vi "Get Call Result.vi"(8 "error in (no error)":errorcluster, 11 "Response body":string) -> (0 "error out":errorcluster, 3 "Call Result":string)   [LabVIEW 2015, in "AWS Core.lvlib"]
uses:
  AWS Core.lvlib
  <vilib>/regexp/Match Regular Expression.xnode
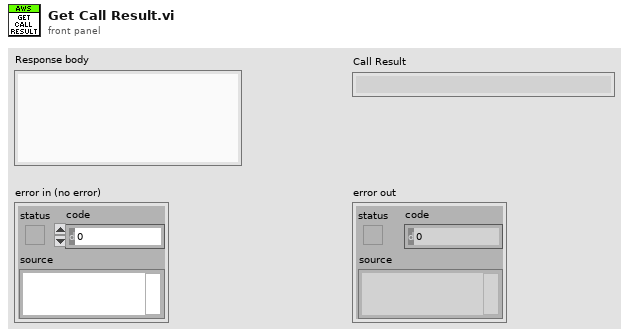
[diagram p1: front panel]
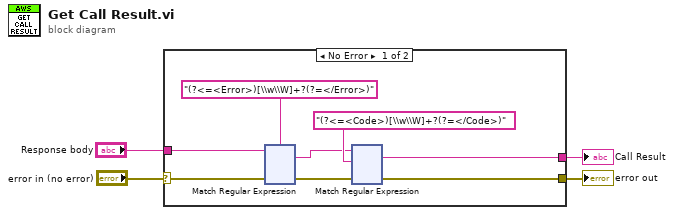
[diagram p0: block diagram]
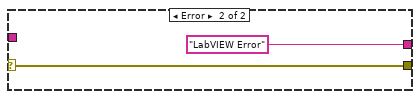
[diagram p2: hidden frame]
diagram:
  n1 = case shown="No Error" "error in (no error)" {
    selector: "error in (no error)" -> [w12 w242]
    tunnel: "Response body" -> [w11 _]
    tunnel: [w7 w242] -> w2
    tunnel: [w5 "LabVIEW Error"] -> w1
    frame No Error {
      n2 = xnode "Match Regular Expression"("input string"=w11, "regular expression"="(?<=<Error>)[\\w\\W]+?(?=</Error>)", "error in"=w12) -> ("whole match"=w6:string, "error out"=w9:errorcluster)  [unwired: 3 in, 3 out]
      n3 = xnode "Match Regular Expression"("input string"=w6, "regular expression"="(?<=<Code>)[\\w\\W]+?(?=</Code>)", "error in"=w9) -> ("whole match"=w5:string, "error out"=w7:errorcluster)  [unwired: 3 in, 3 out]
    }
    frame Error {
    }
  }
  "error out" <- w2
  "Call Result" <- w1
